vi "ManipGroundScore.vi"(2 "Reinit":bool, 3 "Parameter String":string) -> (0 "error out":errorcluster, 1 "Advance Trigger":bool)   [LabVIEW 2020]
doc: "This VI commands the gripper to open or close during a systems check\n\nParameters:\nDecides open or closed state of the gripper (\"open\" or \"close\")"
uses:
  e565341c-ffbe-4def-915a-0842eca45152.vi
  SafeParser_String.vi
  GlobalGripper.vi
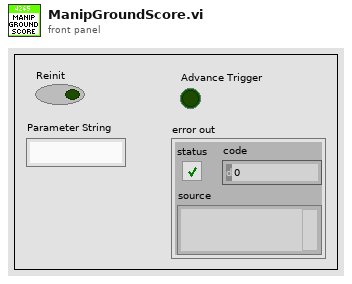
[diagram p1: front panel]
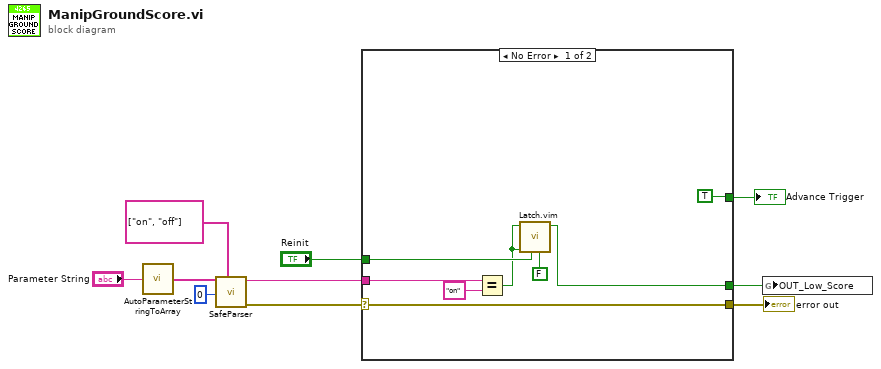
[diagram p0: block diagram]
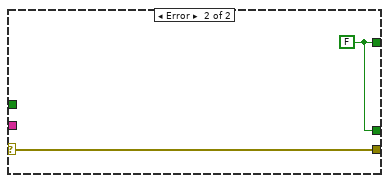
[diagram p2: hidden frame]
diagram:
  n1 = call "AutoParameterStringToArray.vi"("Parameter String"="Parameter String") -> ("Parsed Parameters"=w8:string[])
  n2 = call-poly "SafeParser.vi"("Allowed Values"=string[] ["on", "off"], "Array Index"=0 ("Parameter Index"), "String Array"=w8) -> ("Error Out"=w6:errorcluster, "Typecast Value"=w4:string)  [unwired: 7 in]
  n3 = case shown="No Error" w6 {
    selector: w6 -> [w18 w20]
    tunnel: [w11 w19] -> w2
    tunnel: [w18 w20] -> w5
    tunnel: w4 -> [w17 _]
    tunnel: [TRUE w19] -> w3
    tunnel: "Reinit" -> [w13 _]
    frame No Error {
      n4 = Equal?(x=w17, y="on") -> (x = y?=w12:bool)
      n5 = call "Latch.vim"("Default Value"=FALSE, "Reset"=w13, "Latch Signal"=w12, "Latch Value"=w12) -> ("Latched"=w11:bool)  [unwired: 7 in]
    }
    frame Error {
      w19 = FALSE
    }
  }
  "Advance Trigger" <- w3
  "error out" <- w5
  n6 = global write "GlobalGripper.vi" "OUT_Low_Score"(w2) -> ()
